vi "array H.vi"() -> ()   [LabVIEW 2020]
uses:
  57faaa27-dbc6-406e-82dd-befa86b86c50.vi
  <vilib>/Comparison/Equal/Equal Functor/Equal Functor.lvclass
panel:
  in  "element 4":dbl
  out "index of element":i32
  out "appended array":i32[][](array[numeric])
  out "deleted portion":i32[](array[numeric])
  out "array w/ subset deleted":i32[](array[numeric])
  out "replace supset":i32[](array[numeric])
  out "element 3":i32
  out "element 2":i32
  out "element":i32
  in  "Array 2":i32[][](array[numeric])
  out "size(s) 2":i32[](array[numeric])
  out "size(s)":i32
  in  "Array":i32[](array[numeric])
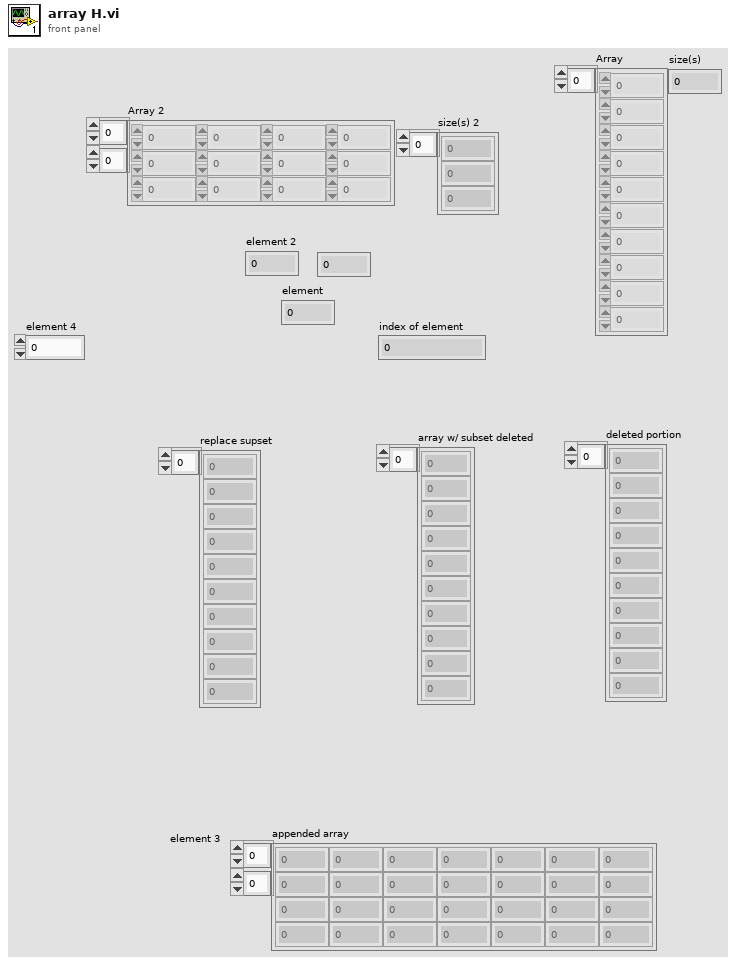
[diagram p1: front panel]
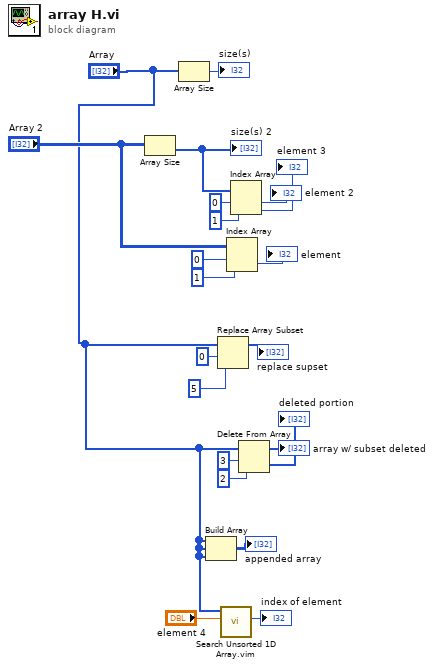
[diagram p0: block diagram]
diagram:
  n1 = Array Size(array="Array 2") -> (size(s)=w17:i32[])
  "size(s) 2" <- w17
  n2 = Array Size(array="Array") -> (size(s)=→"size(s)":i32)
  n3 = Build Array("Array", "Array", "Array") -> (→"appended array":i32[][])
  n4 = Replace Array Subset(array="Array", new element=5 ("new element/subarray"), index=0 ("index (row)")) -> (→"replace supset":i32[])
  n5 = call "Search Unsorted 1D Array.vim"("element"="element 4", "unsorted 1D array"="Array") -> ("index of element"=→"index of element":i32)  [unwired: 9 in]
  n6 = Index Array(array="Array 2", index (row)=0, index (col)=1 ("disabled index (col)")) -> (element=→"element":i32)
  n7 = Index Array(array=w17, index #1=0 ("index"), index #2=1 ("index")) -> (element #1=→"element 2":i32, element #2=→"element 3":i32)
  n8 = Delete From Array(array="Array", length=3, index=2) -> (deleted portion=→"deleted portion":i32[], array with subset deleted=→"array w/ subset deleted":i32[])
